vi "Get Function.vi"(8 "error in (no error)":errorcluster, 11 "result in":refnum<class "result.lvclass">) -> (0 "error out":errorcluster, 2 "function":string, 3 "result out":refnum<class "result.lvclass">)   [LabVIEW 2015, in "result.lvclass"]
uses:
  result.lvclass
  result.lvclass/result.ctl
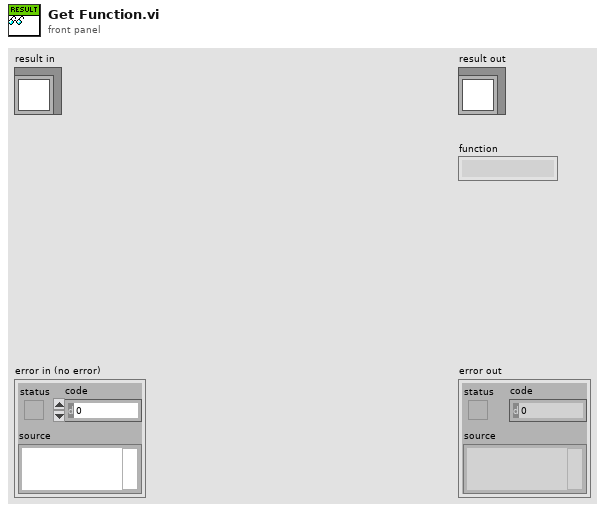
[diagram p1: front panel]
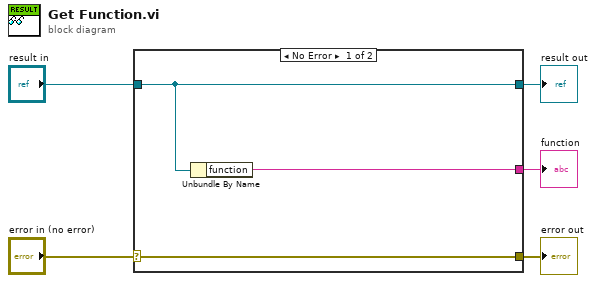
[diagram p0: block diagram]
diagram:
  n1 = case shown="No Error" "error in (no error)" {
    selector: "error in (no error)" -> [w8 w9]
    tunnel: [w8 w9] -> w4
    tunnel: [w7 w10] -> w2
    tunnel: "result in" -> [w7 w10]
    tunnel: [w6 _] -> w1
    frame No Error {
      n2 = Unbundle By Name(w7) -> ("function"=w6:string)
    }
    frame Error {
    }
  }
  "error out" <- w4
  "result out" <- w2
  "function" <- w1
